vi "Main.vi"() -> ()   [LabVIEW 2020]
doc: "Use this template to build a simple state machine design pattern. Each state executes code and determines which state to transition to."
uses:
  controls/File Type.ctl
  controls/State.ctl
  controls/Data.ctl
panel:
  in  "Voltage Acquisition":bool
  in  "File Type":T1
  in  "Open File Location":bool
  in  "Open Data":bool
  in  "Save Data":bool
  out "Current state":string
  out "Data":dbl[](graph)
  in  "Reset Settings":bool
  in  "Clear Graph":bool
  in  "Analyse Data":bool
  in  "Acquire Data":bool
  in  "Configure Data":bool
  in  "Exit":bool
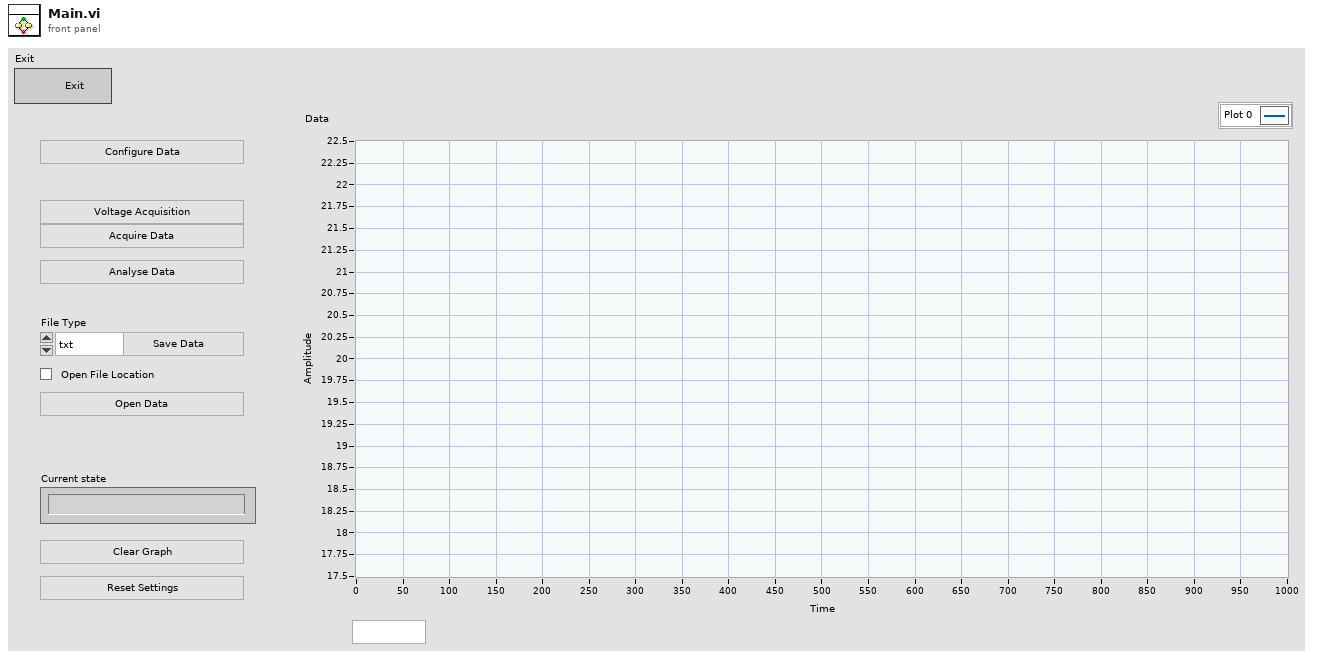
[diagram p1: front panel]
types:
  T1 = typedef "File Type.ctl" = enum16{"txt", "csv", "tdms", ""}
  T2 = typedef "Data.ctl" = cluster{"Configuration Setting":cluster{"offset":dbl, "Signal Type":enum16{"Sine Wave", "Triangle Wave", "Square Wave", "Sawtooth Wave"}, "Amplitude":dbl, "Frequency":dbl, "Phase":dbl, "Noise Amplitude ":dbl}, "Data":dbl[]}
  T3 = typedef "State.ctl" = enum16{"Voltage Acqisition", "Save Data file", "Open Data File", "Initialize", "Wait for Event", "Configure", "Acquire Data State", "Update User interfce", "Reset data", "Clear Data", "Analyse Data", "Stop", "Error"}
  T4 = enum16{"Sine Wave", "Triangle Wave", "Square Wave", "Sawtooth Wave"}
  T5 = cluster{"offset":dbl, "Signal Type":enum16{"Sine Wave", "Triangle Wave", "Square Wave", "Sawtooth Wave"}, "Amplitude":dbl, "Frequency":dbl, "Phase":dbl, "Noise Amplitude ":dbl}
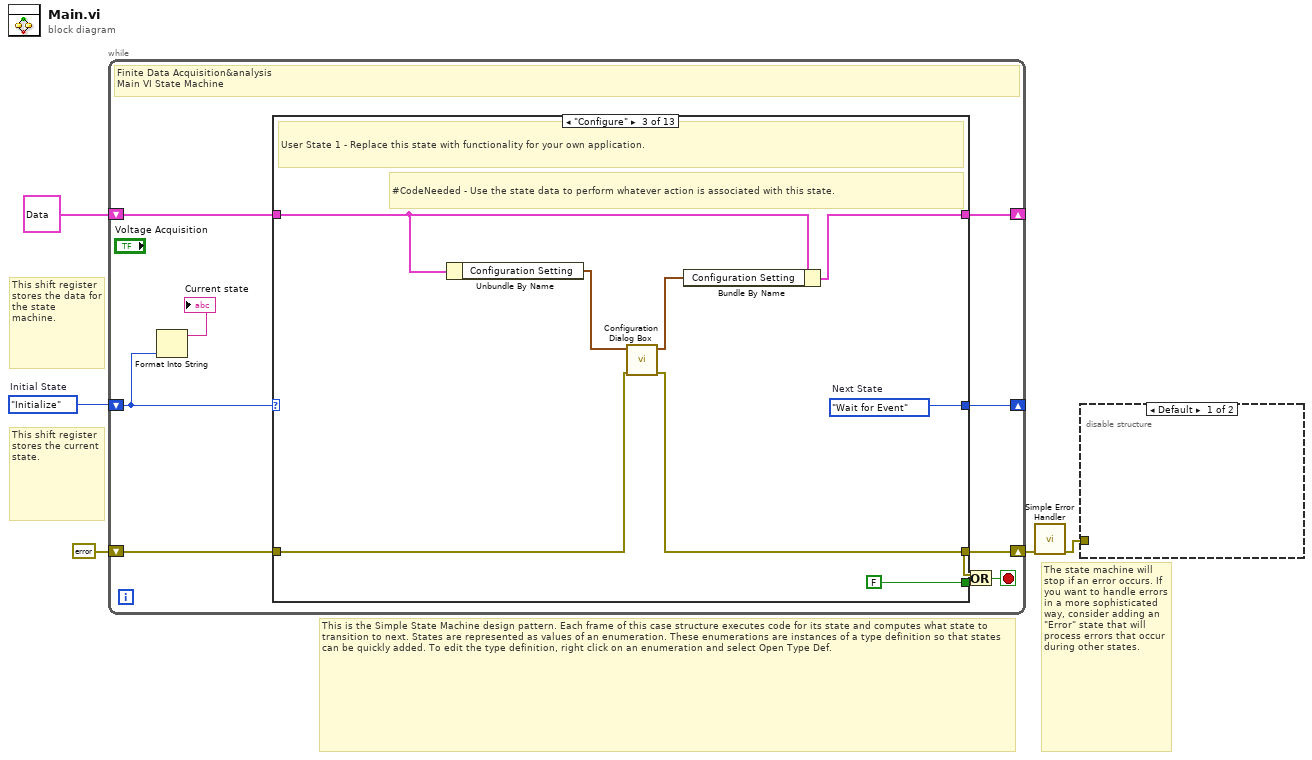
[diagram p0: block diagram]
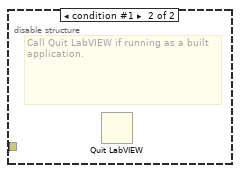
[diagram p2: hidden frame]
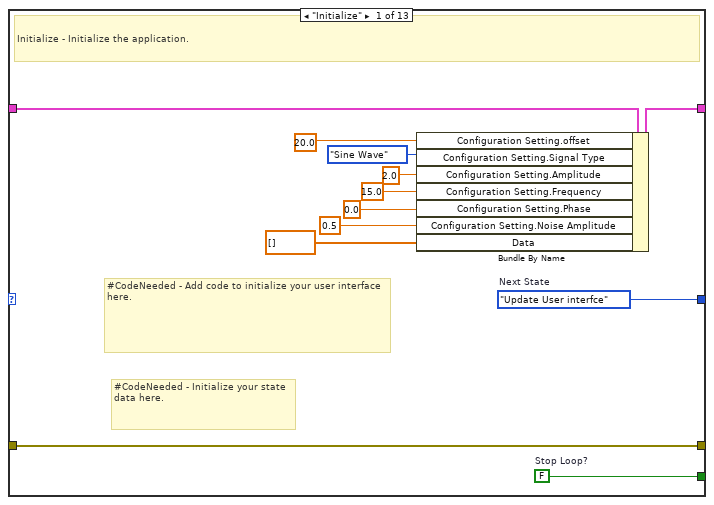
[diagram p3: hidden frame]
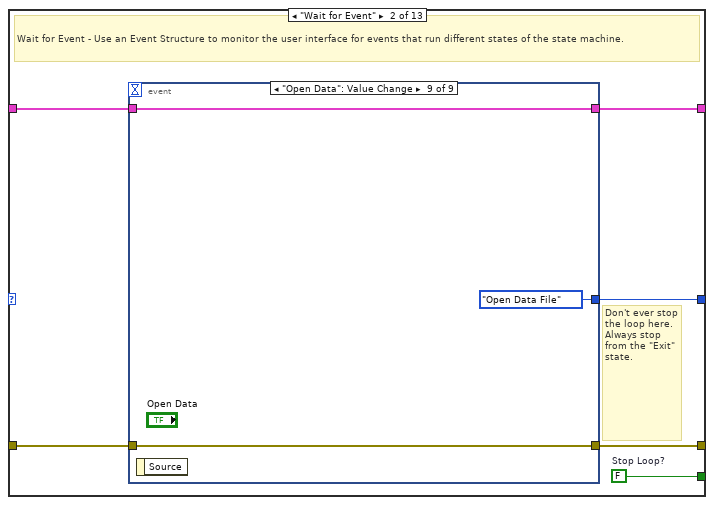
[diagram p4: hidden frame]
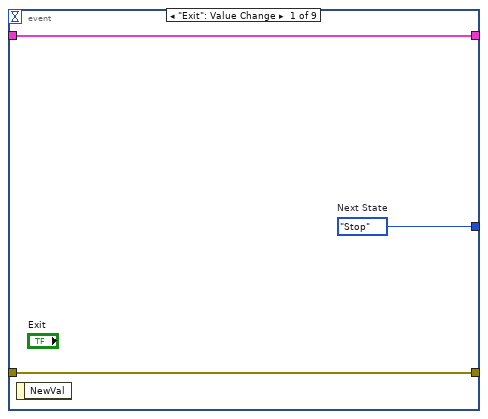
[diagram p5: hidden frame]
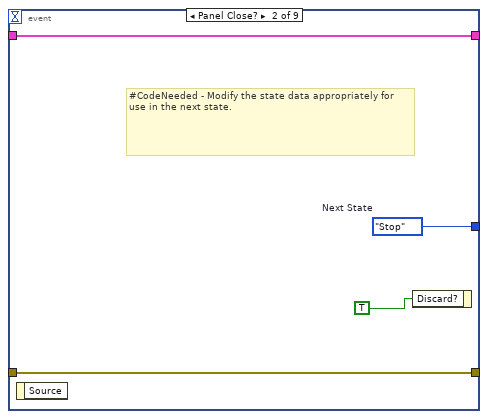
[diagram p6: hidden frame]
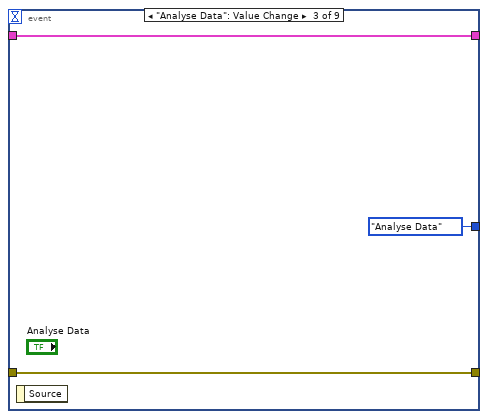
[diagram p7: hidden frame]
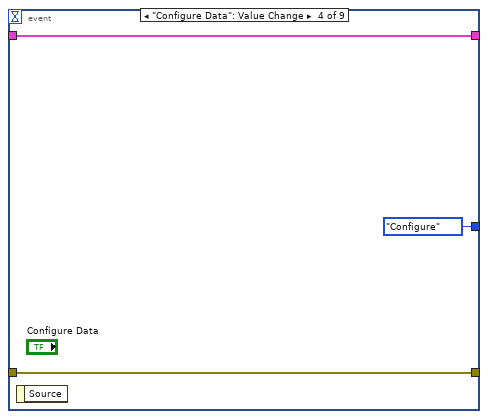
[diagram p8: hidden frame]
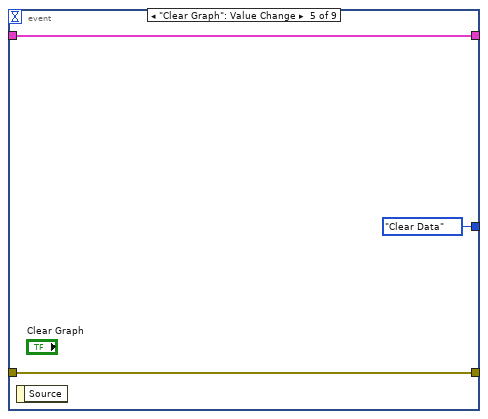
[diagram p9: hidden frame]
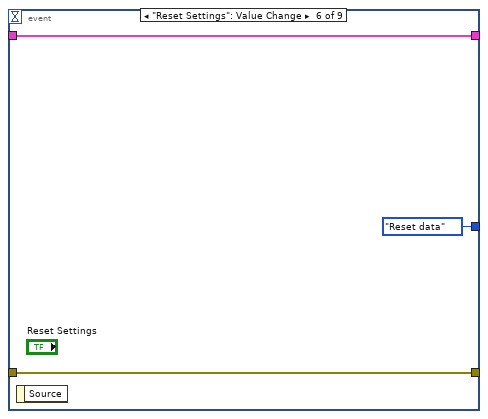
[diagram p10: hidden frame]
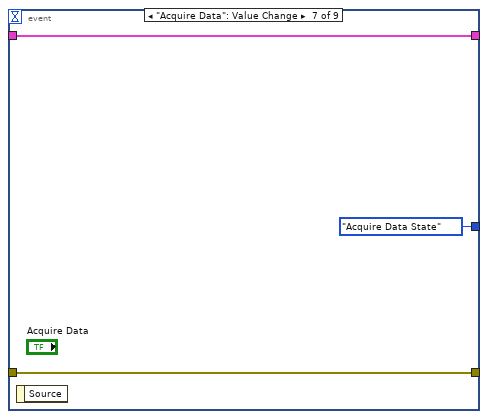
[diagram p11: hidden frame]
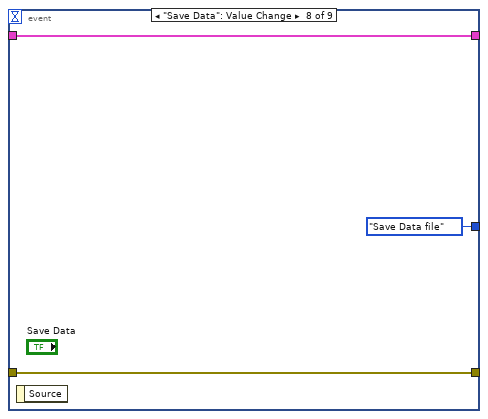
[diagram p12: hidden frame]
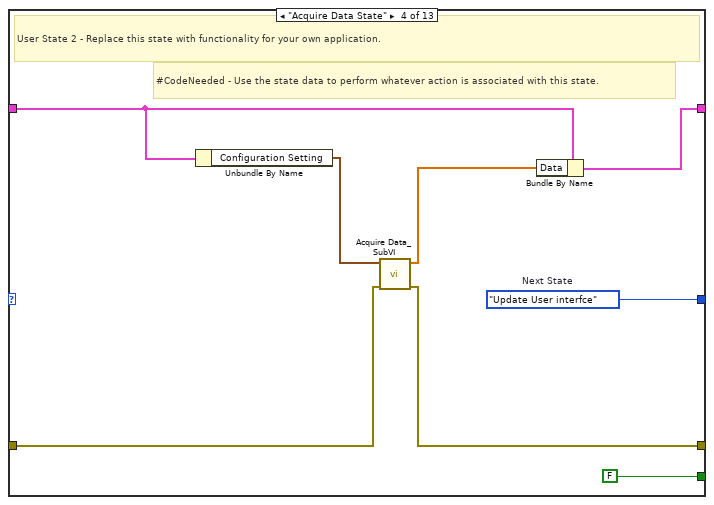
[diagram p13: hidden frame]
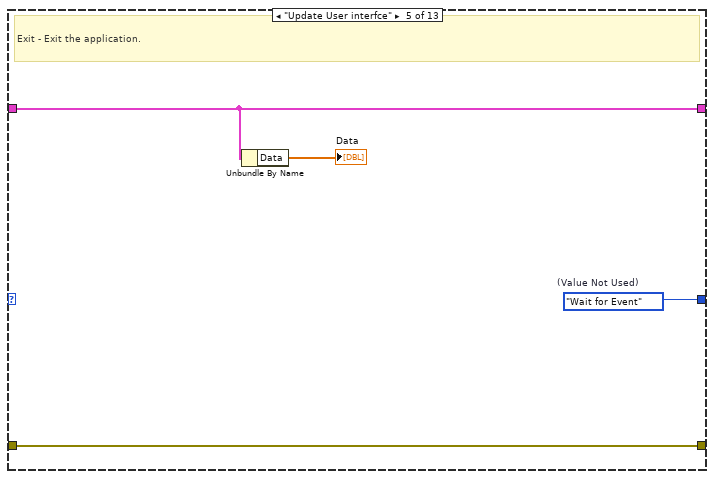
[diagram p14: hidden frame]
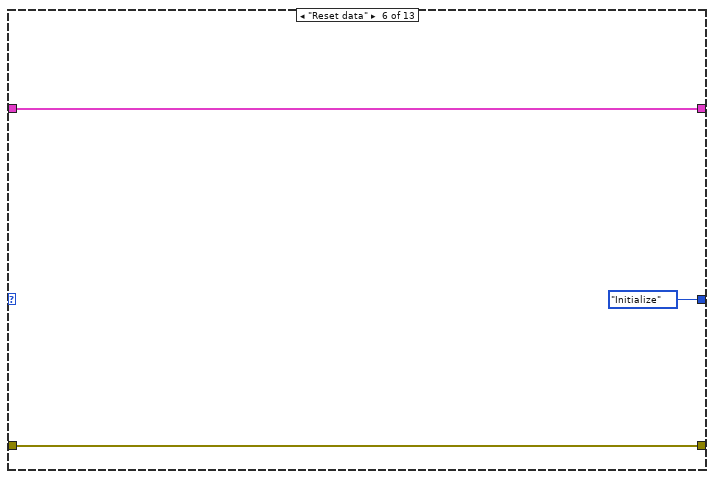
[diagram p15: hidden frame]
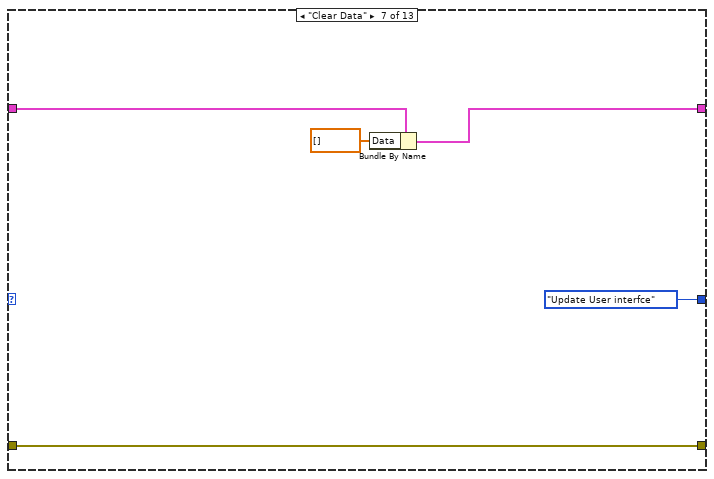
[diagram p16: hidden frame]
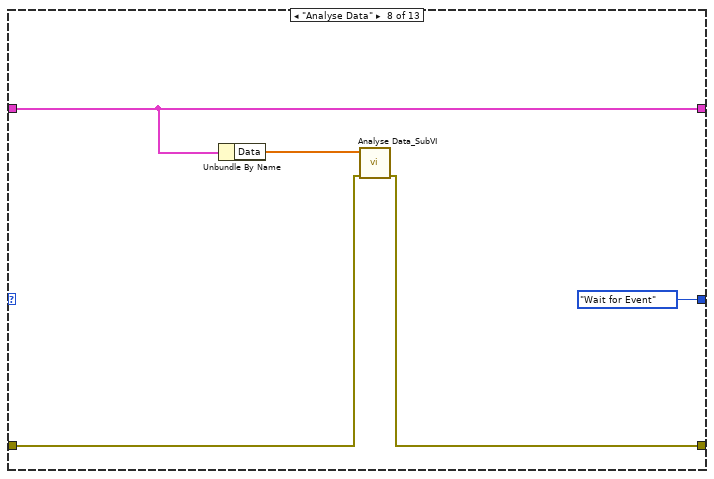
[diagram p17: hidden frame]
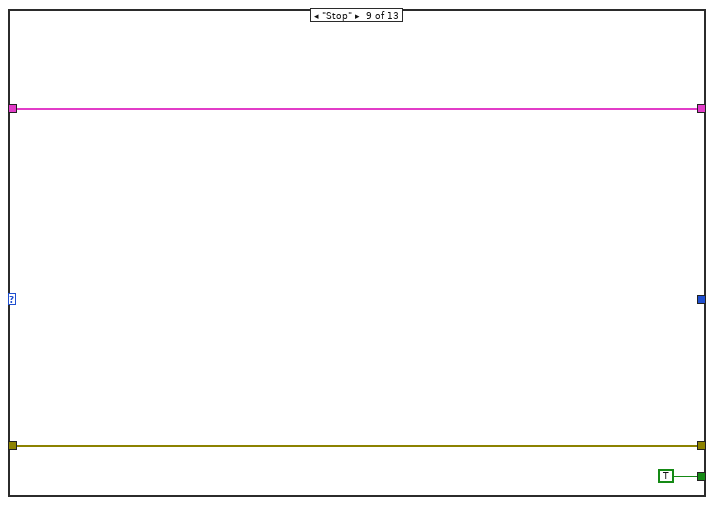
[diagram p18: hidden frame]
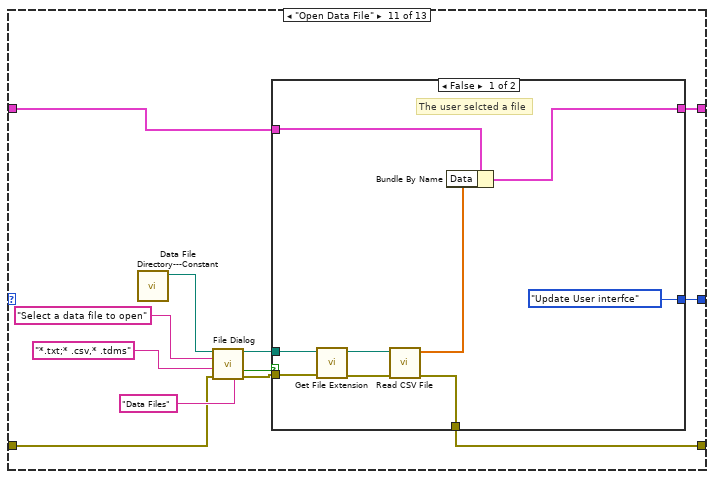
[diagram p20: hidden frame]
diagram:
  w5 = State."Initialize"  # Initial State
  # "The state machine will stop if an error occurs. If you want to handle errors in a more sophisticated way, consider adding an \"Error\" state that will process errors that occur during other states."
  # "This shift register stores the data for the state machine."
  # "This is the Simple State Machine design pattern. Each frame of this case structure executes code for its state and computes what state to transition to next. States are represented as values of an enumeration. These enumerations are instances of a type definition so that states can be quickly added. To edit the type definition, right click on an enumeration and select Open Type Def."
  # "This shift register stores the current state."
  n1 = while {
    shift-right: [w14] -> _
    shift-left: w5 -> [w7]
    shift-right: [w12] -> _
    shift-left: T2 {"Configuration Setting"={"offset"=0.0, "Signal Type"=enum."Sine Wave", "Amplitude"=1.0, "Frequency"=10.0, "Phase"=0.0, "Noise Amplitude "=1.0}, "Data"=[]} ("Data") -> [w13]
    shift-right: [w8] -> w2
    shift-left: errorcluster {"status"=FALSE, "code"=0, "source"=""} ("error constant") -> [w11]
    stop <- w9 stop-if-true
    # "Finite Data Acquisition&analysis \nMain VI State Machine"
    n2 = Format Into String(w7) -> (resulting string=→"Current state":string)  [unwired: 3 in, 1 out]
    n3 = case shown="\"Configure\"" w7 {
      tunnel: [w26 w32 w68 w76 w80 State."Initialize" ("(Value Not Used)") State."Update User interfce" ("(Value Not Used)") State."Wait for Event" ("(Value Not Used)") _ _ w102 State."Wait for Event" ("(Value Not Used)") _] -> w14
      tunnel: [w25 w31 FALSE ("Stop Loop?") FALSE ("Stop Loop?") _ _ _ _ TRUE ("Stop Loop?") _ _ _ _] -> w10
      tunnel: w13 -> [w24 w30 w62 w71 w78 w83 w87 w90 w96 w98 w103 w129 w132]
      tunnel: [w23 w29 w61 w69 w78 w83 w86 w90 w96 w98 w101 w129 w132] -> w12
      tunnel: w11 -> [w22 w28 w66 w74 w79 w82 w88 w92 w95 w97 w104 w124 w131]
      tunnel: [w22 w27 w65 w73 w79 w82 w88 w91 w95 w97 w100 w125 w131] -> w8
      frame "Initialize" {
        w25 = FALSE  # Stop Loop?
        w26 = State."Update User interfce"  # Next State
        # "#CodeNeeded - Initialize your state data here."
        # "#CodeNeeded - Add code to initialize your user interface here."
        # "Initialize - Initialize the application."
        n4 = Bundle By Name(cluster=w24, "Configuration Setting.offset"=20.0, "Configuration Setting.Signal Type"=T4."Sine Wave", "Configuration Setting.Amplitude"=2.0, "Configuration Setting.Frequency"=15.0, "Configuration Setting.Phase"=0.0, "Configuration Setting.Noise Amplitude"=0.5, "Data"=dbl[] []) -> (w23:T2)
      }
      frame "Wait for Event" {
        w31 = FALSE  # Stop Loop?
        # "Don't ever stop the loop here. Always stop from the \"Exit\" state."
        # "Wait for Event - Use an Event Structure to monitor the user interface for events that run different states of the state machine."
        n5 = event shown="[8] \"Open Data\": Value Change" {
          selector: _ -> [_ _ _ _ _ _ _ _ _]
          dyn-events: _ -> [_ _ _ _ _ _ _ _ _]
          timeout: _ -> [_ _ _ _ _ _ _ _ _]
          tunnel: [w35 w39 State."Analyse Data" ("Next State") State."Configure" ("Next State") State."Clear Data" ("Next State") State."Reset data" ("Next State") State."Acquire Data State" ("Next State") State."Save Data file" ("Next State") State."Open Data File" ("Next State")] -> w32
          tunnel: w30 -> [w34 w36 w42 w45 w48 w51 w54 w57 w60]
          tunnel: [w34 w36 w42 w45 w48 w51 w54 w57 w60] -> w29
          tunnel: w28 -> [w33 w38 w41 w44 w47 w50 w53 w56 w59]
          tunnel: [w33 w38 w41 w44 w47 w50 w53 w56 w59] -> w27
          event "Exit": Value Change {
            w35 = State."Stop"  # Next State
            n6 = event-data() -> ()  [unwired: 1 in, 1 out]
          }
          event Panel Close? {
            w39 = State."Stop"  # Next State
            # "#CodeNeeded - Modify the state data appropriately for use in the next state."
            n7 = event-data() -> ()  [unwired: 1 in, 1 out]
            n8 = event-data("Discard?"=TRUE) -> ()  [unwired: 1 in, 1 out]
          }
          event "Analyse Data": Value Change {
            n9 = event-data() -> ()  [unwired: 1 in, 1 out]
          }
          event "Configure Data": Value Change {
            n10 = event-data() -> ()  [unwired: 1 in, 1 out]
          }
          event "Clear Graph": Value Change {
            n11 = event-data() -> ()  [unwired: 1 in, 1 out]
          }
          event "Reset Settings": Value Change {
            n12 = event-data() -> ()  [unwired: 1 in, 1 out]
          }
          event "Acquire Data": Value Change {
            n13 = event-data() -> ()  [unwired: 1 in, 1 out]
          }
          event "Save Data": Value Change {
            n14 = event-data() -> ()  [unwired: 1 in, 1 out]
          }
          event "Open Data": Value Change {
            n15 = event-data() -> ()  [unwired: 1 in, 1 out]
          }
        }
      }
      frame "Configure" {
        w68 = State."Wait for Event"  # Next State
        # "#CodeNeeded - Use the state data to perform whatever action is associated with this state."
        # "User State 1 - Replace this state with functionality for your own application."
        n16 = Unbundle By Name(w62) -> ("Configuration Setting"=w64:T5)
        n17 = call "Configuration Dialog Box.vi"("error in (no error)"=w66, "Configuration Setting In"=w64) -> ("error out"=w65:errorcluster, "Configuration Setting Out"=w63:T5)  [unwired: 8 in]
        n18 = Bundle By Name(cluster=w62, "Configuration Setting"=w63) -> (w61:T2)
      }
      frame "Acquire Data State" {
        w76 = State."Update User interfce"  # Next State
        # "#CodeNeeded - Use the state data to perform whatever action is associated with this state."
        # "User State 2 - Replace this state with functionality for your own application."
        n19 = Unbundle By Name(w71) -> ("Configuration Setting"=w72:T5)
        n20 = call "Acquire Data_SubVI.vi"("error in (no error)"=w74, "Configuration Settings"=w72) -> ("error out"=w73:errorcluster, "Data"=w70:dbl[])  [unwired: 8 in]
        n21 = Bundle By Name(cluster=w71, "Data"=w70) -> (w69:T2)
      }
      frame "Update User interfce" {
        w80 = State."Wait for Event"  # (Value Not Used)
        # "Exit - Exit the application."
        n22 = Unbundle By Name(w78) -> ("Data"=→"Data":dbl[])
      }
      frame "Reset data" {
      }
      frame "Clear Data" {
        n23 = Bundle By Name(cluster=w87, "Data"=dbl[] []) -> (w86:T2)
      }
      frame "Analyse Data" {
        n24 = Unbundle By Name(w90) -> ("Data"=w89:dbl[])
        n25 = call "Analyse Data_SubVI.vi"("error in (no error)"=w92, "Data in"=w89) -> ("error out"=w91:errorcluster)  [unwired: 9 in]
      }
      frame "Stop" {
      }
      frame "Error" {
      }
      frame "Open Data File" {
        n26 = call "Data File Directory---Constant.vi"() -> ("Data File directory"=w107:path)  [unwired: 11 in]
        n27 = call "File Dialog"("start path"=w107, "prompt"="Select a data file to open", "error in"=w104, "pattern (all files)"="*.txt;* .csv,* .tdms", "pattern label"="Data Files") -> ("selected path"=w105:path, "cancelled"=w99:bool, "error out"=w106:errorcluster)  [unwired: 7 in, 1 out]
        n28 = case shown="False" w99 {
          tunnel: w106 -> [w115 w123]
          tunnel: w105 -> [w116 _]
          tunnel: w103 -> [w118 _]
          tunnel: [State."Update User interfce" ("(Value Not Used)") State."Wait for Event" ("(Value Not Used)")] -> w102
          tunnel: [w117 _] -> w101
          tunnel: [w112 w122] -> w100
          frame False {
            # "The user selcted a file"
            n29 = call <vilib>:"Get File Extension.vi"("error in (no error)"=w115, "file"=w116) -> ("error out"=w113:errorcluster, "dup file"=w114:path)  [unwired: 5 in, 3 out]
            n30 = call "Read CSV File.vi"("error in (no error)"=w113, "Path"=w114) -> ("error out"=w112:errorcluster, "Data"=w111:dbl[])  [unwired: 8 in]
            n31 = Bundle By Name(cluster=w118, "Data"=w111) -> (w117:T2)
          }
          frame True {
            n32 = call <vilib>:"Clear Errors.vi"("error in (no error)"=w123, "specific error code to clear (0: all)"=43) -> ("error out"=w122:errorcluster)  [unwired: 4 in, 1 out]
          }
        }
      }
      frame "Save Data file" {
        n33 = Unbundle By Name(w129) -> ("Data"=w127:dbl[])
        n34 = call "Save Data File.vi"("File Type"="File Type", "Data"=w127, "Open File Location"="Open File Location", "error in (no error)"=w124) -> ("error out"=w125:errorcluster)  [unwired: 6 in]
      }
      frame "Voltage Acqisition" {
      }
    }
    n35 = Or(x=w8, y=w10) -> (x .or. y?=w9:bool)
  }
  n36 = call <vilib>:"Simple Error Handler.vi"("error in (no error)"=w2) -> ("error out"=w1:errorcluster)  [unwired: 4 in, 4 out]
  n37 = disable-structure shown="Default" {
    disable-tunnel: w1 -> [_ _]
    frame condition #0 (active) {
    }
    frame condition #1 {
      # "Call Quit LabVIEW if running as a built application."
      n38 = Quit LabVIEW() -> ()  [unwired: 1 in]
    }
  }
